vi "Vi Caller Is top level.vi"() -> (3 "Caller is top level":bool)   [LabVIEW 2009]
doc: "Determines if the current vi's caller is top level? Uses call chain.\nThis vi is reentrant"
panel:
  out "call chain":string[](array[string])
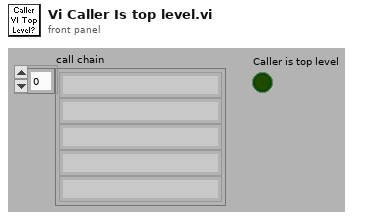
[diagram p1: front panel]
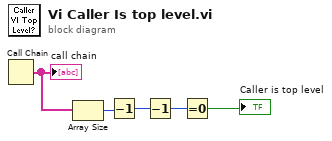
[diagram p0: block diagram]
diagram:
  n1 = Call Chain() -> (call chain=w5:string[])
  "call chain" <- w5
  n2 = Array Size(array=w5) -> (size(s)=w4:i32)
  n3 = Decrement(x=w4) -> (x-1=w2:i32)
  n4 = Decrement(x=w2) -> (x-1=w1:i32)
  n5 = Equal To 0?(x=w1) -> (x = 0?=→"Caller is top level":bool)
